vi "OMV_Snap.vi"(8 "error in (no error)":errorcluster, 11 "VISA Refnum in":refnum<visa-resource-name>) -> (0 "error out":errorcluster, 2 "image data":T1, 3 "VISA Refnum out":refnum<visa-resource-name>)   [LabVIEW 2017]
uses:
  <vilib>/picture/picture.llb/imagedata.ctl
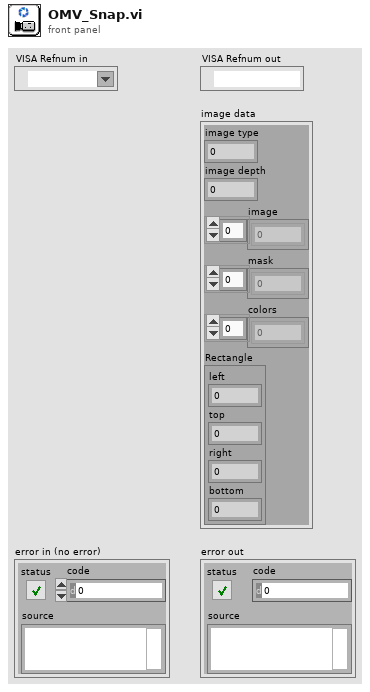
[diagram p1: front panel]
types:
  T1 = typedef "imagedata.ctl" = cluster{"image type":i32, "image depth":i32, "image":u8[], "mask":u8[], "colors":u32[], "Rectangle":cluster{"left":i16, "top":i16, "right":i16, "bottom":i16}}
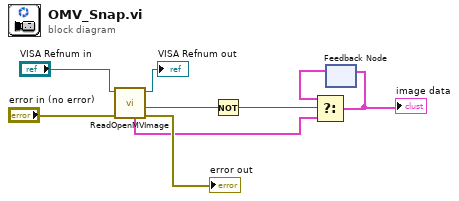
[diagram p0: block diagram]
diagram:
  n1 = call "ReadOpenMVImage.vi"("error in"="error in (no error)", "VISA Refnum in"="VISA Refnum in") -> ("error out"=→"error out":errorcluster, "Good?"=w2:bool, "VISA Refnum out"=→"VISA Refnum out":refnum<visa-resource-name>, "image data"=w4:T1)  [unwired: 4 in, 2 out]
  n2 = Not(x=w2) -> (.not. x?=w1:bool)
  n3 = feedback #1() -> (w3:T1)  [unwired: 1 in]
  n4 = Select(t=w3, s=w1, f=w4) -> (s? t:f=w6:T1)
  "image data" <- w6
  n5 = feedback-in #1(w6) -> ()
